vi "resetPosition.vi"(11 "Device in":refnum<k24>) -> (3 "Device out":refnum<k24>)   [LabVIEW 2014]
doc: "André Romero - 2018\nandretec@ifsc.usp.br\n\nReset counter position"
uses:
  C:/user-Lab/AndreTec/GITs/andretec/Thorlabs-Vector-Move/kinesisTec/Kinesis/Thorlabs.MotionControl.TCube.DCServoCLI.dll
  kinesisTec/Kinesis/Thorlabs.MotionControl.TCube.DCServoCLI.dll
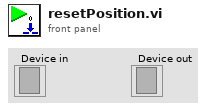
[diagram p1: front panel]
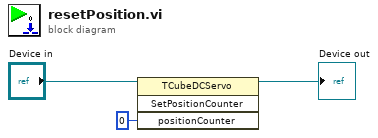
[diagram p0: block diagram]
diagram:
  n1 = invoke class="TCubeDCServo" method="SetPositionCounter"(reference="Device in", "positionCounter"=0) -> (reference out=→"Device out":refnum<k24>)  [unwired: 2 in, 3 out]
